vi "Test.vi"() -> ()   [LabVIEW 2012]
uses:
  Opening Purpose.ctl
panel:
  out "Image":T1(plugin-control)
  out "Number of Pages":i32
  out "error out":errorcluster
  in  "Original File Path":path
  in  "Opening Purpose":T2
  in  "TIFF File Path":path
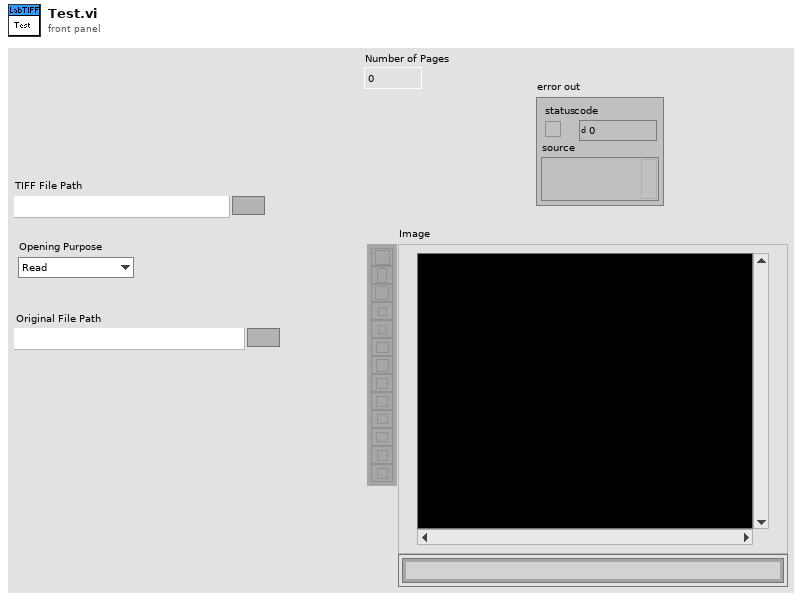
[diagram p1: front panel]
types:
  T1 = typedef "IMAQ Image.ctl" = refnum<image>
  T2 = typedef "Opening Purpose.ctl" = enum16{"Read", "Write"}
  T3 = typedef "Image Type" = u32
  T4 = enum16{"8 bit unsigned", "16 bit unsigned", "16 bit signed", "32 bit float"}
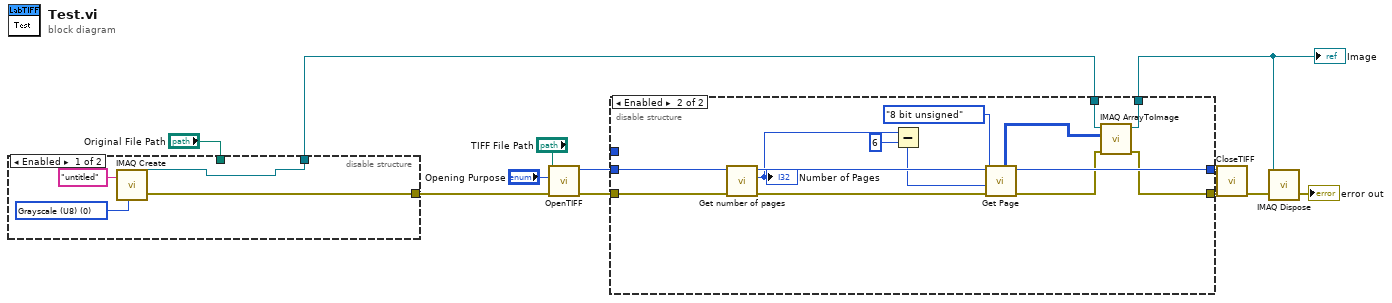
[diagram p0: block diagram]
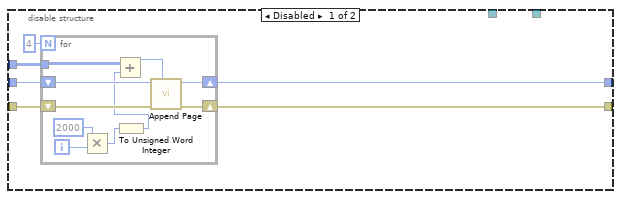
[diagram p2: hidden frame]
diagram:
  n1 = disable-structure shown="Enabled" {
    disable-tunnel: "Original File Path" -> [_ _]
    disable-tunnel: [w13 _] -> w9
    disable-tunnel: [w14 _] -> w2
    frame Enabled {
      w15 = T3 0 items=["Grayscale (U8)", "Grayscale (I16)", "Grayscale (SGL)", "Complex (CSG)", "RGB (U32)", "HSL (U32)", "RGB (U64)", "Grayscale (U16)"] ("Image Type")
      n2 = call "IMAQ Create"("Image Name"="untitled", "Image Type"=w15) -> ("New Image"=w14:T1, "error out"=w13:errorcluster)  [unwired: 3 in]
    }
    frame Disabled {
    }
  }
  n3 = call "OpenTIFF.vi"("error in (no error)"=w9, "Opening Purpose"="Opening Purpose", "File Path"="TIFF File Path") -> ("error out"=w8:errorcluster, "TIFF File Ref"=w7:i32)  [unwired: 7 in]
  n4 = disable-structure shown="Enabled" {
    disable-tunnel: w8 -> [w22 w45]
    disable-tunnel: w7 -> [w21 w46]
    disable-tunnel: [w20 w42] -> w6
    disable-tunnel: [w19 w34] -> w5
    disable-tunnel: _ -> [w18 _]
    disable-tunnel: w2 -> [_ w37]
    disable-tunnel: [_ w36] -> w1
    frame Disabled {
      n5 = for {
        N: 4 -> [_]
        tunnel: w18 -> [w26]
        shift-right: [w30] -> w19
        shift-left: w22 -> [w32]
        shift-right: [w31] -> w20
        shift-left: w21 -> [w27]
        i -> [w29]
        n6 = Multiply(x=2000, y=w29) -> (x*y=w25:i32)
        n7 = To Unsigned Word Integer(number=w25) -> (unsigned 16bit integer=w24:u16)
        n8 = Add(x=w26, y=w24) -> (x+y=w23:u16)
        n9 = call "Append Page.vi"("U16 Image"=w23, "error in (no error)"=w32, "TIFF File Ref"=w27) -> ("error out"=w30:errorcluster, "TIFF File Ref out"=w31:i32)  [unwired: 7 in]
      }
    }
    frame Enabled {
      n10 = call "Get number of pages.vi"("error in (no error)"=w45, "TIFF File ref"=w46) -> ("error out"=w43:errorcluster, "Number of Pages"=w41:i32, "TIFF File ref out"=w44:i32)  [unwired: 7 in]
      "Number of Pages" <- w41
      n11 = Subtract(x=w41, y=6) -> (x-y=w39:i32)
      n12 = call "Get Page.vi"("error in (no error)"=w43, "Frame number"=w39, "Type of Image"=T4."8 bit unsigned", "TIFF File Ref"=w44) -> ("error out"=w35:errorcluster, "TIFF File Ref out"=w42:i32, "U8 Image out"=w33:u8[][])  [unwired: 2 in, 3 out]
      n13 = call "IMAQ ArrayToImage"("error in (no error)"=w35, "Image Pixels (U8)"=w33, "Image"=w37) -> ("error out"=w34:errorcluster, "Image Out"=w36:T1)  [unwired: 7 in]
    }
  }
  "Image" <- w1
  n14 = call "CloseTIFF.vi"("error in (no error)"=w5, "TIFF File Ref"=w6) -> ("error out"=w4:errorcluster)  [unwired: 9 in]
  n15 = call "IMAQ Dispose"("Image"=w1, "error in (no error)"=w4) -> ("error out"=→"error out":errorcluster)  [unwired: 4 in]
